vi "Configure Calender.vi"(0 "VISA resource name":refnum<visa-resource-name>, 5 "First Weekday (0: Sunday)":u16(ring) items=["Sunday", "Monday"], 11 "error in (no error)":errorcluster) -> (4 "VISA resource name out":refnum<visa-resource-name>, 15 "error out":errorcluster)   [LabVIEW 2020, in "Yokogawa GX Series.lvlib"]
doc: "Sets the calendar display format.\n\nCommand: SCalFormat\n\nNote: This VI does nothing when the instrument is GM10."
uses:
  <instrlib>/Yokogawa GX Series/Yokogawa GX Series.lvlib
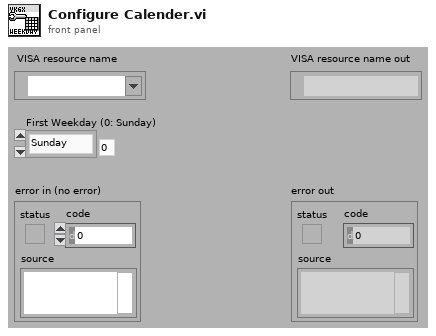
[diagram p1: front panel]
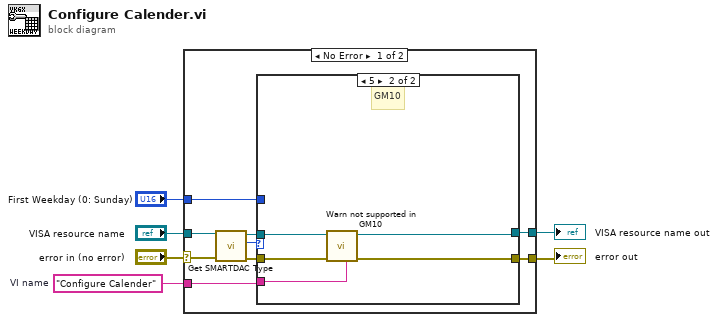
[diagram p0: block diagram]
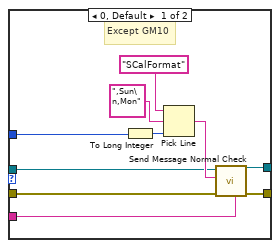
[diagram p2: hidden frame]
diagram:
  w5 = "Configure Calender"  # VI name
  n1 = case shown="No Error" "error in (no error)" {
    selector: "error in (no error)" -> [w10 w31]
    tunnel: "VISA resource name" -> [w11 w32]
    tunnel: w5 -> [w15 _]
    tunnel: [w14 w32] -> w4
    tunnel: [w13 w31] -> w3
    tunnel: "First Weekday (0: Sunday)" -> [w12 _]
    frame No Error {
      n2 = call <instrlib>:"Get SMARTDAC Type.vi"("error in (no error)"=w10, "VISA resource name"=w11) -> ("error out"=w8:errorcluster, "SMARTDAC+ Type"=w7:u16, "VISA resource name out"=w9:refnum<visa-resource-name>)  [unwired: 7 in]
      n3 = case shown="5" w7 {
        tunnel: w15 -> [w25 w26]
        tunnel: [w24 w28] -> w14
        tunnel: [w23 w27] -> w13
        tunnel: w12 -> [w17 _]
        tunnel: w9 -> [w19 w30]
        tunnel: w8 -> [w18 w29]
        frame 0, Default {
          # "Except GM10"
          n4 = To Long Integer(number=w17) -> (32bit integer=w16:i32)
          n5 = Pick Line(string ("")="SCalFormat", multi-line string=",Sun\n,Mon", line index=w16) -> (output string=w20:string)
          n6 = call <instrlib>:"Send Message Normal Check.vi"("Source (\"\")"=w25, "error in (no error)"=w18, "Send Message (\"\")"=w20, "VISA resource name"=w19) -> ("error out"=w23:errorcluster, "VISA resource name out"=w24:refnum<visa-resource-name>)  [unwired: 2 in, 4 out]
        }
        frame 5 {
          # "GM10"
          n7 = call <instrlib>:"Warn not supported in GM10.vi"("Source (\"\")"=w26, "error in (no error)"=w29, "VISA resource name"=w30) -> ("error out"=w27:errorcluster, "VISA resource name out"=w28:refnum<visa-resource-name>)  [unwired: 7 in]
        }
      }
    }
    frame Error {
    }
  }
  "error out" <- w3
  "VISA resource name out" <- w4
